vi "Write address.vi"(8 "error in (no error)":errorcluster, 10 "address":string="localhost", 11 "TCP_Client in":refnum<class "TCP_Client.lvclass">) -> (0 "error out":errorcluster, 3 "TCP_Client out":refnum<class "TCP_Client.lvclass">)   [LabVIEW 2018, in "TCP_Client.lvlib" / "TCP_Client.lvclass"]
uses:
  TCP_Client.lvclass
  TCP_Client.lvclass/TCP_Client.ctl
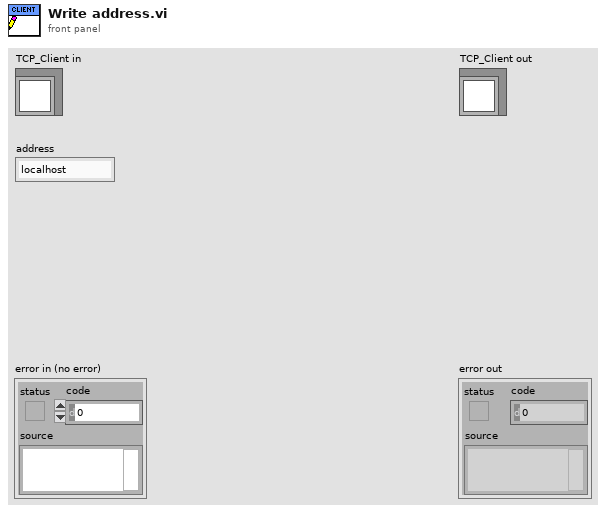
[diagram p1: front panel]
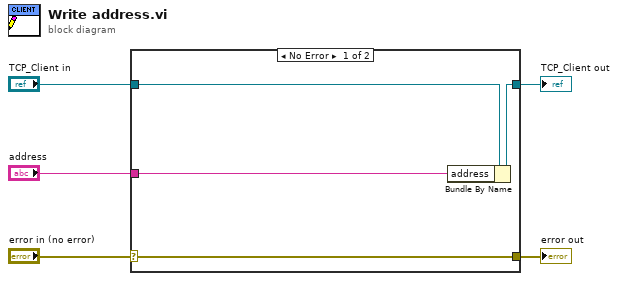
[diagram p0: block diagram]
diagram:
  n1 = case shown="No Error" "error in (no error)" {
    selector: "error in (no error)" -> [w9 w10]
    tunnel: [w9 w10] -> w4
    tunnel: [w7 w11] -> w2
    tunnel: "TCP_Client in" -> [w8 w11]
    tunnel: "address" -> [w6 _]
    frame No Error {
      n2 = Bundle By Name(cluster=w8, "address"=w6) -> (w7:refnum<class "TCP_Client.lvclass">)
    }
    frame Error {
    }
  }
  "error out" <- w4
  "TCP_Client out" <- w2
